vi "Get Display Name and Relative Path.vi"(8 "error in (no error)":errorcluster, 10 "Library":string, 11 "Destination Path":path) -> (0 "error out":errorcluster, 2 "Relative Path":string, 3 "Display Name":string)   [LabVIEW 2021, in "CIF Build Actions.lvlib"]
uses:
  CIF Build Actions.lvlib
  CIFCore/Common/Typedef/Errors.ctl
  <vilib>/CIF Foundation/CIF Utilities/Errors/Append Error Location.vi
  <vilib>/Utility/LVLibp/NI_PackedLibraryUtility.lvlib
  CIFCore/Common/CIFCoreCommon.lvlib
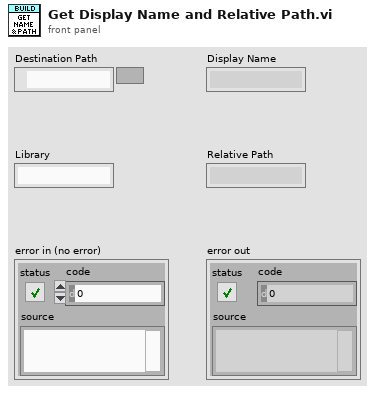
[diagram p1: front panel]
types:
  T1 = typedef "CIFCoreCommon.lvlib/Errors.ctl" = enum16{"Invalid Clock ID", "Long Sleep", "gRPC Server Not Found", "Config Parse", "Timestamp Wrap", "Delayed Execution", "Duplicate Channel", "Missing Channel", "Incorrect Type", "Flatten Error", "Unflatten Data", "Unique Name", "Plugin Not Found", "Plugin Type Not Found", "Plugin Version Not Found", "Manager Not Found", "Numerical Issue", "Time Jump", "Clock ID Match", "Channel Length", "Plugin Connection", "gRPC Server Connection", "PPL Name Match", "Build", "Config Log Parse", "Plugin Load", "UI Subpanel Load", "Python Name", "Invalid Name"}
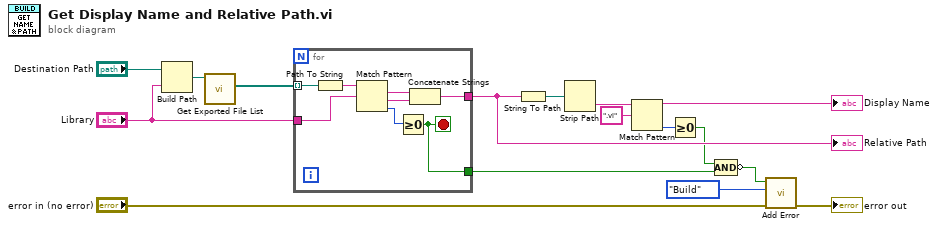
[diagram p0: block diagram]
diagram:
  n1 = Build Path(base path="Destination Path", name or relative path="Library") -> (appended path=w11:path)
  n2 = call <vilib>:"Get Exported File List.vi"("packed library path"=w11) -> ("paths"=w14:path[])  [unwired: 8 in, 2 out]
  n3 = for {
    tunnel: w14 -> [w24] mode=indexing
    tunnel: "Library" -> [w22]
    tunnel: [w18] -> w9
    tunnel: [w17] -> w6
    stop <- w17 stop-if-true
    n4 = Path To String(path=w24) -> (string=w23:string)
    n5 = Match Pattern(string=w23, regular expression=w22) -> (match substring=w21:string, after substring=w20:string, offset past match=w19:i32)  [unwired: 1 in, 1 out]
    n6 = Greater Or Equal To 0?(x=w19) -> (x >= 0?=w17:bool)
    n7 = Concatenate Strings(w21, w20) -> (w18:string)
  }
  "Relative Path" <- w9
  n8 = String To Path(string=w9) -> (path=w10:path)
  n9 = Strip Path(path=w10) -> (name=w8:string)  [unwired: 1 out]
  n10 = Match Pattern(string=w8, regular expression=".vi") -> (before substring=→"Display Name":string, offset past match=w7:i32)  [unwired: 1 in, 2 out]
  n11 = Greater Or Equal To 0?(x=w7) -> (x >= 0?=w5:bool)
  n12 = Compound Arithmetic op=AND(w5, w6) -> (invert w3:bool)
  n13 = call "Add Error.vi"("error in (no error)"="error in (no error)", "Error"=Errors."Build", "Insert Error"=w3) -> ("error out"=→"error out":errorcluster)  [unwired: 8 in]
